vi "Throw Channel Overlap Error.vi"(7 "error source vi name":string, 8 "error in (no error)":errorcluster, 10 "current channel block":T1={"string offset"=0, "string data type"=enum."Bool", "engine data type"=enum."Bool", "name"="", "settings"=[], "units"="V"} {"string offset" format="%d bytes"}, 11 "previous channel block":T1={"string offset"=0, "string data type"=enum."Bool", "engine data type"=enum."Bool", "name"="", "settings"=[], "units"="V"} {"string offset" format="%d bytes"}) -> (0 "error out":errorcluster)   [LabVIEW 2017, in "DSF Core.lvlib" / "Configuration Session.lvclass"]
uses:
  Configuration Session.lvclass
  Typedefs/DSF Engine Channel Configuration.ctl
  Typedefs/DSF Data Type.ctl
  Typedefs/DSF Settings Info.ctl
  <vilib>/NI/Memory Manager/Static Errors.lvlib
  <vilib>/NI/Memory Manager/VIs/Write Numeric Scalar to Source (Base10 U64).vi
  Framework/Framework.lvclass
  Errors.ctl
  DSF Core.lvlib
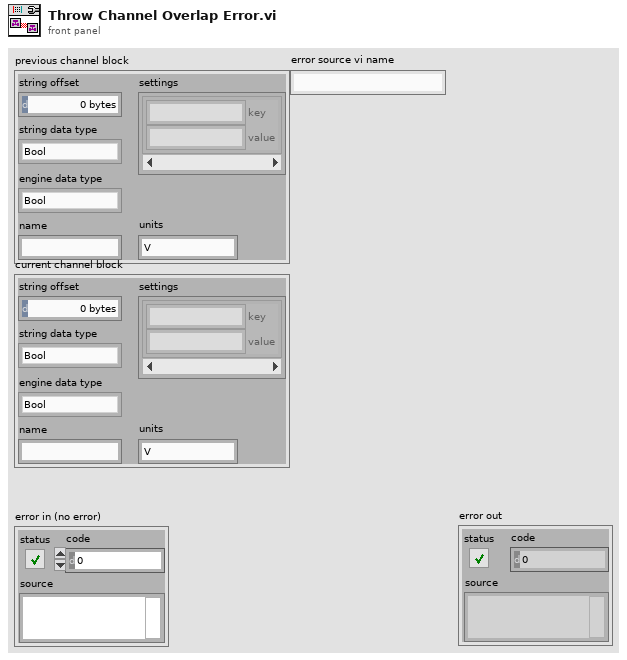
[diagram p1: front panel]
types:
  T1 = typedef "DSF Core.lvlib/DSF Engine Channel Configuration.ctl" = cluster{"string offset":u64, "string data type":T2, "engine data type":T2, "name":string, "settings":T3, "units":string}
  T2 = typedef "DSF Core.lvlib/DSF Data Type.ctl" = enum8{"Bool", "SGL", "DBL", "I8", "I16", "I32", "I64", "U8", "U16", "U32", "U64"}
  T3 = typedef "DSF Core.lvlib/DSF Settings Info.ctl" = cluster{"key":string, "value":string}[]
  T4 = typedef "DSF Core.lvlib/Configuration Session.lvclass/Errors.ctl" = enum16{"Channel Overlap", "Invalid Engine Offset", "Invalid JSON"}
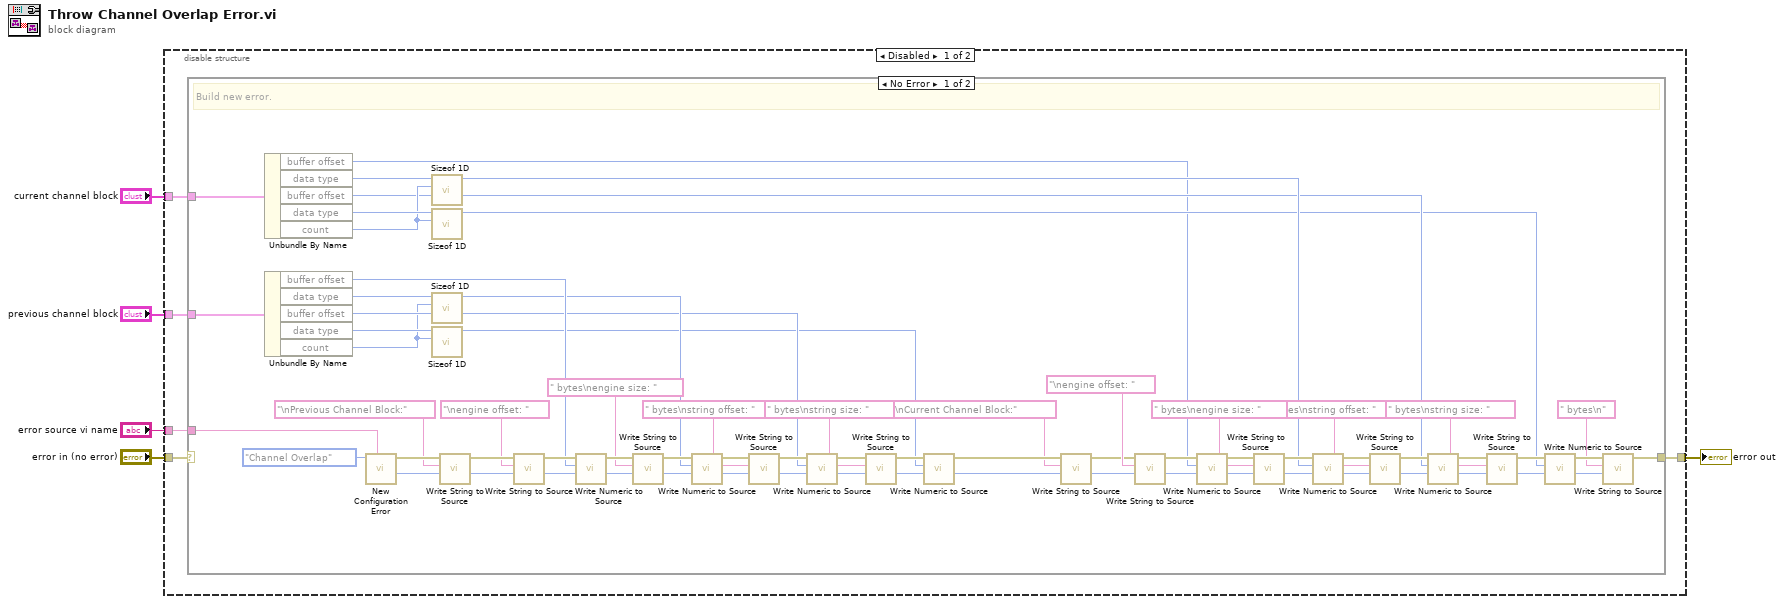
[diagram p0: block diagram]
diagram:
  n1 = disable-structure shown="Disabled" {
    disable-tunnel: "error in (no error)" -> [w10 w80]
    disable-tunnel: [w9 w80] -> w4
    disable-tunnel: "error source vi name" -> [w8 _]
    disable-tunnel: "previous channel block" -> [w7 _]
    disable-tunnel: "current channel block" -> [w6 _]
    frame Disabled {
      n2 = case shown="No Error" w10 {
        selector: w10 -> [_ w79]
        tunnel: [w13 w79] -> w9
        tunnel: w8 -> [w77 _]
        tunnel: w7 -> [w74 _]
        tunnel: w6 -> [w67 _]
        frame No Error {
          # "Build new error."
          n3 = Unbundle By Name(w67) -> ("buffer offset"=w11:u64, "data type"=w44:T2, "buffer offset"=w18:u64, "data type"=w43:T2, "count"=w42:u64)
          n4 = Unbundle By Name(w74) -> ("buffer offset"=w66:u64, "data type"=w63:T2, "buffer offset"=w53:u64, "data type"=w52:T2, "count"=w51:u64)
          n5 = call "New Configuration Error.vi"("error source vi name"=w77, "configuration error"=Errors."Channel Overlap") -> ("new offset"=w75:i32, "error out"=w76:errorcluster)  [unwired: 8 in]
          n6 = call "Sizeof 1D.vi"("count"=w42, "data type"=w44) -> ("size in bytes"=w19:u64)  [unwired: 9 in]
          n7 = call "Sizeof 1D.vi"("count"=w42, "data type"=w43) -> ("size in bytes"=w17:u64)  [unwired: 9 in]
          n8 = call "Sizeof 1D.vi"("count"=w51, "data type"=w63) -> ("size in bytes"=w59:u64)  [unwired: 9 in]
          n9 = call "Sizeof 1D.vi"("count"=w51, "data type"=w52) -> ("size in bytes"=w45:u64)  [unwired: 9 in]
          n10 = call <vilib>:"Write String to Source.vi"("offset"=w75, "string"="\nPrevious Channel Block:", "error in"=w76) -> ("new offset"=w70:i32, "error out"=w72:errorcluster)  [unwired: 7 in]
          n11 = call <vilib>:"Write String to Source.vi"("offset"=w70, "string"="\nengine offset: ", "error in"=w72) -> ("new offset"=w68:i32, "error out"=w69:errorcluster)  [unwired: 7 in]
          n12 = call-poly <vilib>:"Write Numeric to Source.vi"("offset"=w68, "value"=w66, "error in"=w69) -> ("new offset"=w64:i32, "error out"=w65:errorcluster)  [unwired: 7 in]
          n13 = call <vilib>:"Write String to Source.vi"("offset"=w64, "string"=" bytes\nengine size: ", "error in"=w65) -> ("new offset"=w60:i32, "error out"=w61:errorcluster)  [unwired: 7 in]
          n14 = call-poly <vilib>:"Write Numeric to Source.vi"("offset"=w60, "value"=w59, "error in"=w61) -> ("new offset"=w57:i32, "error out"=w58:errorcluster)  [unwired: 7 in]
          n15 = call <vilib>:"Write String to Source.vi"("offset"=w57, "string"=" bytes\nstring offset: ", "error in"=w58) -> ("new offset"=w54:i32, "error out"=w55:errorcluster)  [unwired: 7 in]
          n16 = call-poly <vilib>:"Write Numeric to Source.vi"("offset"=w54, "value"=w53, "error in"=w55) -> ("new offset"=w47:i32, "error out"=w48:errorcluster)  [unwired: 7 in]
          n17 = call <vilib>:"Write String to Source.vi"("offset"=w47, "string"=" bytes\nstring size: ", "error in"=w48) -> ("new offset"=w50:i32, "error out"=w49:errorcluster)  [unwired: 7 in]
          n18 = call-poly <vilib>:"Write Numeric to Source.vi"("offset"=w50, "value"=w45, "error in"=w49) -> ("new offset"=w20:i32, "error out"=w21:errorcluster)  [unwired: 7 in]
          n19 = call <vilib>:"Write String to Source.vi"("offset"=w20, "string"=" bytes\n\nCurrent Channel Block:", "error in"=w21) -> ("new offset"=w24:i32, "error out"=w22:errorcluster)  [unwired: 7 in]
          n20 = call <vilib>:"Write String to Source.vi"("offset"=w24, "string"="\nengine offset: ", "error in"=w22) -> ("new offset"=w26:i32, "error out"=w25:errorcluster)  [unwired: 7 in]
          n21 = call-poly <vilib>:"Write Numeric to Source.vi"("offset"=w26, "value"=w11, "error in"=w25) -> ("new offset"=w28:i32, "error out"=w27:errorcluster)  [unwired: 7 in]
          n22 = call <vilib>:"Write String to Source.vi"("offset"=w28, "string"=" bytes\nengine size: ", "error in"=w27) -> ("new offset"=w31:i32, "error out"=w30:errorcluster)  [unwired: 7 in]
          n23 = call-poly <vilib>:"Write Numeric to Source.vi"("offset"=w31, "value"=w19, "error in"=w30) -> ("new offset"=w33:i32, "error out"=w32:errorcluster)  [unwired: 7 in]
          n24 = call <vilib>:"Write String to Source.vi"("offset"=w33, "string"=" bytes\nstring offset: ", "error in"=w32) -> ("new offset"=w36:i32, "error out"=w35:errorcluster)  [unwired: 7 in]
          n25 = call-poly <vilib>:"Write Numeric to Source.vi"("offset"=w36, "value"=w18, "error in"=w35) -> ("new offset"=w40:i32, "error out"=w39:errorcluster)  [unwired: 7 in]
          n26 = call <vilib>:"Write String to Source.vi"("offset"=w40, "string"=" bytes\nstring size: ", "error in"=w39) -> ("new offset"=w37:i32, "error out"=w38:errorcluster)  [unwired: 7 in]
          n27 = call-poly <vilib>:"Write Numeric to Source.vi"("offset"=w37, "value"=w17, "error in"=w38) -> ("new offset"=w15:i32, "error out"=w14:errorcluster)  [unwired: 7 in]
          n28 = call <vilib>:"Write String to Source.vi"("offset"=w15, "string"=" bytes\n", "error in"=w14) -> ("error out"=w13:errorcluster)  [unwired: 7 in, 1 out]
        }
        frame Error {
          # "Incoming error. Pass through."
        }
      }
    }
    frame Enabled {
    }
  }
  "error out" <- w4
